vi "LookForPreInstHold.vi"(4 "Home reward":cluster{"Fix":dbl, "Rnd":dbl}={"Fix"=0.5, "Rnd"=0.5} {"Rnd" format="%.4f"; "Fix" format="%_4g"}, 5 "Home reward?":bool, 6 "DI Task":refnum<k21>, 7 "Touch lines":T2={"Home touch"=0, "Touch 1"=1, "Touch 2"=2, "Touch 3"=3, "Touch 4"=4}, 8 "Touching home\nlast time?":bool, 9 "Just initialized\nhold loop?":bool, 10 "Composite time":dbl format="%.4f", 11 "DO Task":refnum<k21>="BlueSimple_DO") -> (0 "Touching home\nthis time?":bool, 1 "Just initialized\nhold loop out?":bool, 3 "Next stage in trial":T1(ring))   [LabVIEW 2010]
panel:
  # "+"
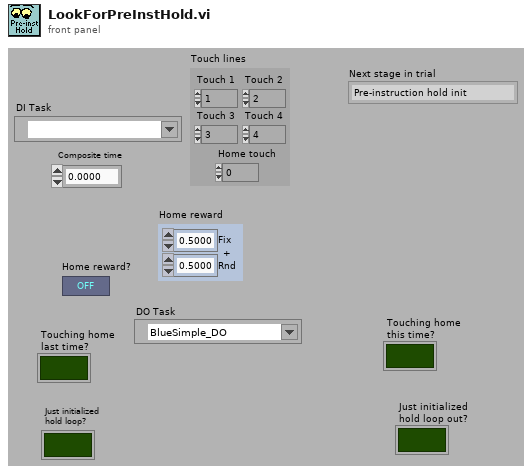
[diagram p1: front panel]
types:
  T1 = enum16{"Pre-instruction hold init", "Pre-instruction hold", "Instruction init", "Instruction", "Post-instruction hold init", "Post-instruction hold", "Target capture init", "Target capture", "Target hold init", "Target hold", "Reward stage", "Intertrial"}
  T2 = cluster{"Home touch":i16, "Touch 1":i16, "Touch 2":i16, "Touch 3":i16, "Touch 4":i16}
  T3 = enum16{"Home", "Touch 1", "Touch 2", "Touch 3", "Touch 4", "None"}
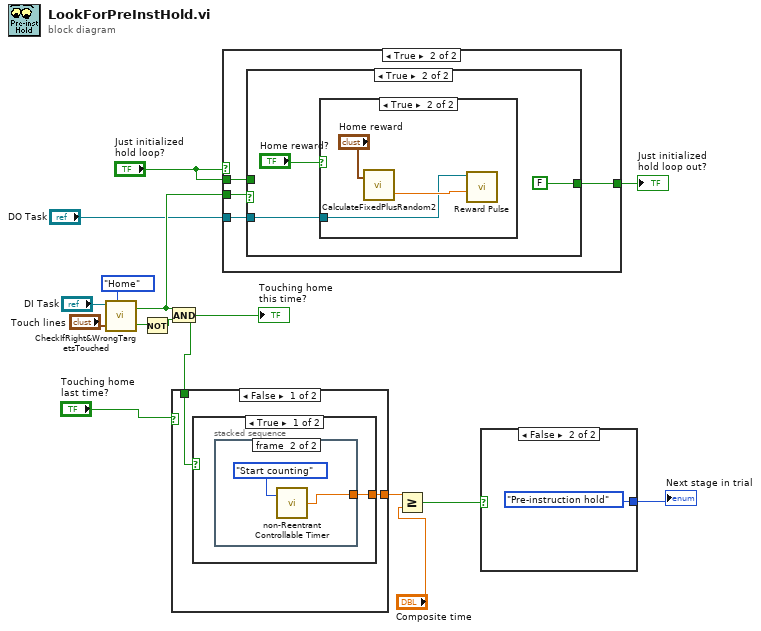
[diagram p0: block diagram]
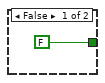
[diagram p2: hidden frame]
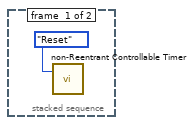
[diagram p5: hidden frame]
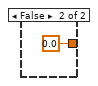
[diagram p6: hidden frame]
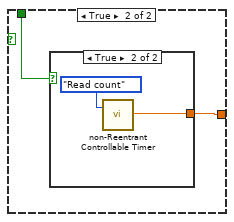
[diagram p7: hidden frame]
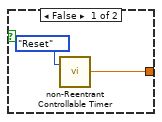
[diagram p8: hidden frame]
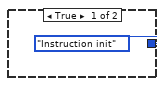
[diagram p9: hidden frame]
diagram:
  n1 = call "CheckIfRight&WrongTargetsTouched.vi"("Target"=T3."Home", "Touch sensor lines"="Touch lines", "DI Task"="DI Task") -> ("Wrong target touched?"=w12:bool, "Target touched?"=w5:bool)  [unwired: 3 in]
  n2 = Not(x=w12) -> (.not. x?=w11:bool)
  n3 = And(x=w5, y=w11) -> (x .and. y?=w9:bool)
  "Touching home\nthis time?" <- w9
  n4 = case shown="False" "Touching home\nlast time?" {
    tunnel: w9 -> [w17 w24]
    tunnel: [w16 w23] -> w13
    frame False {
      n5 = case shown="True" w17 {
        tunnel: [w18 0.0 ("Time out")] -> w16
        frame True {
          n6 = stacked-sequence {
            tunnel: [_ w21] -> w18
            frame #0 {
              n7 = call "non-Reentrant Controllable Timer.vi"("Enum"=enum16{"Start counting", "Read count", "Reset"}."Reset") -> ()  [unwired: 1 in, 1 out]
            }
            frame #1 {
              n8 = call "non-Reentrant Controllable Timer.vi"("Enum"=enum16{"Start counting", "Read count", "Reset"}."Start counting") -> ("Time out"=w21:dbl)  [unwired: 1 in]
            }
          }
        }
        frame False {
        }
      }
    }
    frame True {
      n9 = case shown="True" w24 {
        tunnel: [w25 w27] -> w23
        frame False {
          n10 = call "non-Reentrant Controllable Timer.vi"("Enum"=enum16{"Start counting", "Read count", "Reset"}."Reset") -> ("Time out"=w25:dbl)  [unwired: 1 in]
        }
        frame True {
          n11 = call "non-Reentrant Controllable Timer.vi"("Enum"=enum16{"Start counting", "Read count", "Reset"}."Read count") -> ("Time out"=w27:dbl)  [unwired: 1 in]
        }
      }
    }
  }
  n12 = case shown="True" "Just initialized\nhold loop?" {
    tunnel: w5 -> [_ w33]
    tunnel: [FALSE w32] -> w4
    tunnel: "Just initialized\nhold loop?" -> [_ w31]
    tunnel: "DO Task" -> [_ w30]
    frame False {
    }
    frame True {
      n13 = case shown="True" w33 {
        tunnel: [w34 FALSE ("Just initialized\nhold loop out?")] -> w32
        tunnel: w31 -> [w34 _]
        tunnel: w30 -> [_ w35]
        frame False {
        }
        frame True {
          n14 = case shown="True" "Home reward?" {
            tunnel: w35 -> [_ w38]
            frame False {
            }
            frame True {
              n15 = call "CalculateFixedPlusRandom2.vi"("Component times"="Home reward") -> ("time in ms"=w39:dbl)  [unwired: 1 in, 1 out]
              n16 = call "Reward Pulse.vi"("Pulse duration (ms)"=w39, "DO Task"=w38) -> ()  [unwired: 8 in]
            }
          }
        }
      }
    }
  }
  "Just initialized\nhold loop out?" <- w4
  n17 = Greater Or Equal?(x=w13, y="Composite time") -> (x >= y?=w15:bool)
  n18 = case shown="False" w15 {
    tunnel: [T1."Instruction init" ("Current stage") T1."Pre-instruction hold" ("Current stage")] -> w6
    frame True {
    }
    frame False {
    }
  }
  "Next stage in trial" <- w6
